vi "TryUpdateAnalogInputSample.vi"   [LabVIEW 2018]
uses:
  <vilib>/Platform/TimedLoop/XDataNode/timing_clust.ctl
  <vilib>/Platform/TimedLoop/XDataNode/nitl_modes.ctl
  <vilib>/Platform/TimedLoop/XDataNode/wakeup.ctl
  Telemetry/TelemetryDataTypes.ctl
  Telemetry/TelemetryUpdateModes.ctl
  Telemetry/TelemetryFields.ctl
  <vilib>/rvi/Emulation/niFpgaEmulationIsFPGAContextNoSignature.vi
  <vilib>/rvi/Emulation/niFpgaSctlEmulationGetInTimedLoop.vi
  <vilib>/rvi/errors/niFpgaSetErrorForExecOnDevCompSimple.vi
  <vilib>/rvi/eio/common/nirviEmuReportErrorAndStop.vi
  <vilib>/rvi/DataTransferAndStorage/Container/Common/niFpgaContainerGetUniqueNameForEmu.vi
  <vilib>/rvi/FIFO/Fifo_Resource/nirvififoEmulationSetSize.vi
  <vilib>/rvi/FIFO/Fifo_Resource/nirviFifoEmulationQueueMgr.vi
  <instcachedir>/0/nirviFifoEmulationQueueMgr_E5CAEC123FF24DC58D834DCA3CDAA9B5.lvgen/nirviFifoEmulationQueueMgr_E5CAEC123FF24DC58D834DCA3CDAA9B5_025.vi
  <vilib>/Utility/error.llb/Clear Errors.vi
  <vilib>/rvi/FIFO/Fifo_Resource/nirvififoEmulationCreateLock.vi
  <vilib>/rvi/Emulation/niFpgaProcessEmulError.vi
  <vilib>/rvi/FIFO/Fifo_Resource/nirvififoEmulationObtainLock.vi
  <vilib>/rvi/FIFO/Fifo_Resource/nirvififoEmulationReleaseLock.vi
  <vilib>/rvi/occurrence/nirviWaitOnOccurrenceBase.vi
  <vilib>/rvi/errors/nirviReportUnexpectedCaseInternalError.vi
  <vilib>/rvi/errors/nirviReportUnexpectedCaseInternalError (U32).vi
  <vilib>/rvi/Emulation/niFpgaEmulationReportErrorSimple.vi
  <vilib>/rvi/Emulation/niFpgaGetClockAttributes.vi
  <vilib>/rvi/Emulation/niFpgaCriticalErrorInLSC.vi
  <instcachedir>/0/nirviFifoEmulationQueueMgr_E5CAEC123FF24DC58D834DCA3CDAA9B5.lvgen/nirviFifoEmulationQueueMgr_E5CAEC123FF24DC58D834DCA3CDAA9B5_022.vi
  <vilib>/rvi/FIFO/Fifo_Resource/nirvififoEmulationDetermineInputValidOut.vi
  <instcachedir>/0/nirviFifoEmulationQueueMgr_E5CAEC123FF24DC58D834DCA3CDAA9B5.lvgen/nirviFifoEmulationQueueMgr_E5CAEC123FF24DC58D834DCA3CDAA9B5_023.vi
  <vilib>/rvi/Memory/Memory_Emulation/niFpgaMemoryEmulationCacheClearOnFirstRun.vi
  <vilib>/rvi/Memory/Memory_Emulation/nirvimemoryEmulationManagerCache_MakeExclusive.vi
  <vilib>/rvi/Memory/Memory_Emulation/niFpgaMemoryEmulationValidateCache.vi
  <vilib>/rvi/Memory/Memory_Emulation/nirvimemoryEmulationManagerCache_InsertValue.vi
  <vilib>/rvi/Memory/Memory_Emulation/nirvimemoryEmulationManagerCache_ReleaseExclusive.vi
  <vilib>/rvi/Memory/Memory_Emulation/nirvimemoryEmulationManagerCache_GetValue.vi
  <vilib>/rvi/Memory/Memory_Emulation/nirvimemoryEmulationManagerCache_SetValue.vi
  <instcachedir>/0/nirviFifoEmulationQueueMgr_E5CAEC123FF24DC58D834DCA3CDAA9B5.lvgen/nirviFifoEmulationQueueMgr_E5CAEC123FF24DC58D834DCA3CDAA9B5_002.vi
  <vilib>/rvi/DataTransferAndStorage/Container/XNode/niFpgaContainer.xnode
  <vilib>/rvi/FIFO/Fifo_Resource/nirvififoEmulationRead.vi
  <vilib>/Platform/TimedLoop/XDataNode/XDataNode.xnode
  <vilib>/rvi/FIFO/Fifo_Resource/nirvififoEmulationWrite.vi
  <vilib>/rvi/DataTransferAndStorage/Register/Emulation/niFpgaRegisterEmulation.vi
  <vilib>/Platform/TimedLoop/XDataNode/XDNodeRunTimeDep.lvlib
types:
  T1 = cluster{"Sample":u64, "Timestamp":u64, "Raw1":sgl, "Raw2":sgl, "Raw3":sgl, "Raw4":sgl, "Raw5":sgl, "Raw6":sgl, "Raw7":sgl, "Raw8":sgl, "Raw9":sgl, "Raw10":sgl, "Raw11":sgl, "Raw12":sgl, "Raw13":sgl, "Raw14":sgl, "Raw15":sgl, "Raw16":sgl}
  T2 = typedef "TelemetryFields.ctl" = enum16{"None", "AnalogInputSampleCount", "AnalogInputSampleTimestamp", "AnalogInputRaw1", "AnalogInputRaw2", "AnalogInputRaw3", "AnalogInputRaw4", "AnalogInputRaw5", "AnalogInputRaw6", "AnalogInputRaw7", "AnalogInputRaw8", "AnalogInputRaw9", "AnalogInputRaw10", "AnalogInputRaw11", "AnalogInputRaw12", "AnalogInputRaw13", "AnalogInputRaw14", "AnalogInputRaw15", "AnalogInputRaw16", "DigitalInputSampleCount", "DigitalInputSampleTimestamp", "DigitalInputStates", "ThermocoupleSampleCount", "ThermocoupleSampleTimestamp", "ThermocoupleRaw1", "ThermocoupleRaw2", "ThermocoupleRaw3", "ThermocoupleRaw4", "ThermocoupleRaw5", "ThermocoupleRaw6", "ThermocoupleRaw7", "ThermocoupleRaw8", "ThermocoupleRaw9", "ThermocoupleRaw10", "ThermocoupleRaw11", "ThermocoupleRaw12", "ThermocoupleRaw13", "ThermocoupleRaw14", "ThermocoupleRaw15", "ThermocoupleRaw16", "WindSensorTxBytes", "WindSensorTxFrames", "WindSensorRxBytes", "WindSensorRxFrames", "WindSensorErrorTimestamp", "WindSensorErrorCode", "WindSensorSampleTimestamp", "WindSensorXRaw", "WindSensorYRaw", "WindSensorZRaw", "WindSensorSonicTempRaw", "WindSensorDiagWord", "WindSensorRecordCount", "FlowSensorTxBytes", "FlowSensorTxFrames", "FlowSensorRxBytes", "FlowSensorRxFrames", "FlowSensorErrorTimestamp", "FlowSensorErrorCode", "FlowSensorSampleTimestamp", "FlowSensorSignalStrength", "FlowSensorFlowRate", "FlowSensorNetTotalizer", "FlowSensorPositiveTotalizer", "FlowSensorNegativeTotalizer", "FlowSensorTemperature1", "FlowSensorTemperature2", "VFDTxBytes", "VFDTxFrames", "VFDRxBytes", "VFDRxFrames", "VFDErrorTimestamp", "VFDErrorCode", "VFDSampleTimestamp", "VFDVelocityBits", "VFDDiagnosticCode", "VFDFrequencyCommand", "VFDOutputFrequency", "VFDOutputCurrent", "VFDDCBusVoltage", "VFDOutputVoltage"}
  T3 = typedef "TelemetryUpdateModes.ctl" = enum8{"=", "+", "-", "|"}
  T4 = typedef "TelemetryDataTypes.ctl" = enum8{"U8", "U16", "U32", "U64", "I8", "I16", "I32", "I64", "SGL"}
  T5 = typedef "XDNodeRunTimeDep.lvlib/timing_clust.ctl" = cluster{"Expected End [f-1]":u64, "Actual End [f-1]":u64, "Finished Late? [f-1]":bool, "Expected End [i-1]":u64, "Actual End [i-1]":u64, "Finished Late? [i-1]":bool, "Expected Start [i]":u64, "Actual Start [i]":u64, "Expected Start [f]":u64, "Actual Start [f]":u64, "Source Name":string, "Structure Name":string, "Period":i64, "Deadline":i64, "Offset":i64, "Start":i64, "Priority":i32, "Timeout":i32, "Mode":T6, "Wakeup Reason":T7, "Error":errorcluster, "Source Type":string, "Secondary Source Type":string, "Global End Time":u64, "Global Start Time":u64, "Frame Duration":u64, "Iteration Duration":u64, "Assigned CPU":i32, "I/O Scan Engine Mode":u32}
  T6 = typedef "XDNodeRunTimeDep.lvlib/nitl_modes.ctl" = enum32{"No Change", "Process missed periods, maintain original phase", "Discard missed periods, maintain original phase", "Process missed periods, ignore original phase", "Discard missed periods, ignore original phase"}
  T7 = typedef "XDNodeRunTimeDep.lvlib/wakeup.ctl" = enum32{"Normal", "Aborted", "Asynchronous wakeup", "Timing source error", "Timed loop error", "Timeout"}
  T8 = typedef "TelemetryUpdateData.ctl" = cluster{"DataType":T4, "Mode":T3, "Field":T2, "Data":u64}
  T9 = typedef "TelemetryUpdateDataSGL.ctl" = cluster{"Mode":T3, "Field":T2, "Data":sgl}
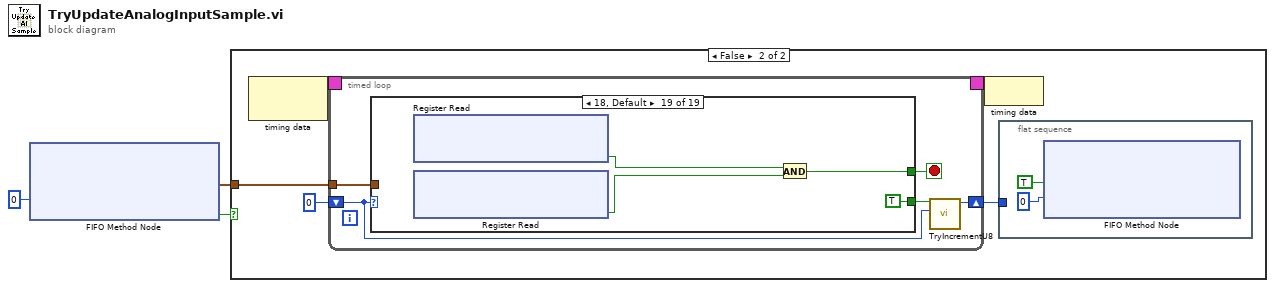
[diagram p0: block diagram]
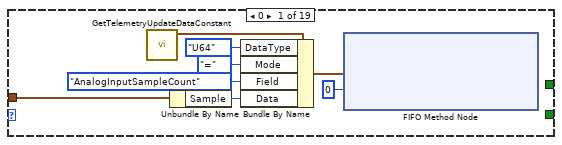
[diagram p3: hidden frame]
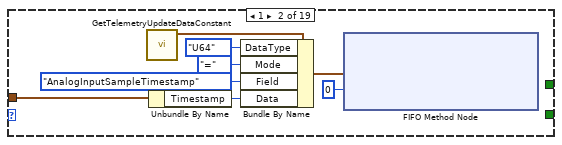
[diagram p4: hidden frame]
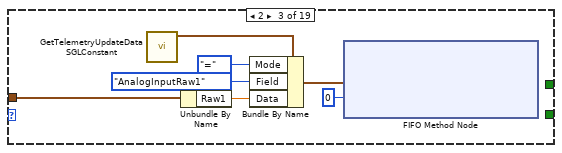
[diagram p5: hidden frame]
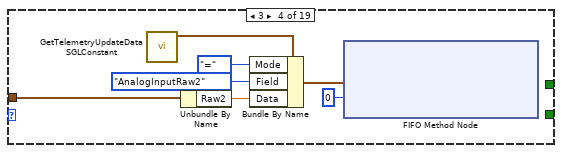
[diagram p6: hidden frame]
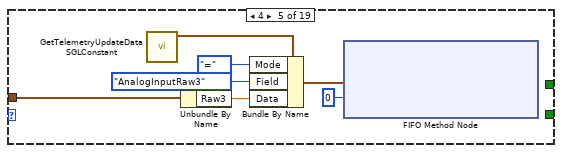
[diagram p7: hidden frame]
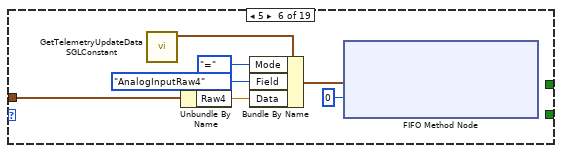
[diagram p8: hidden frame]
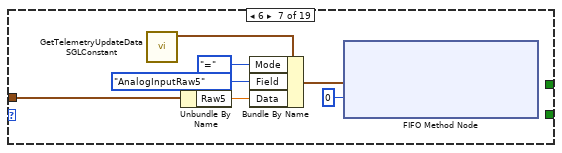
[diagram p9: hidden frame]
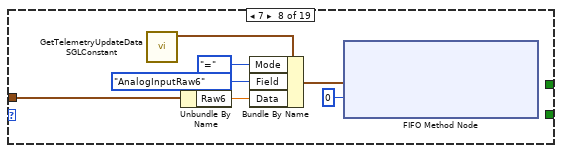
[diagram p10: hidden frame]
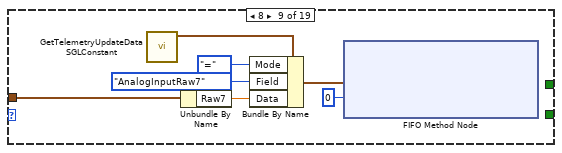
[diagram p11: hidden frame]
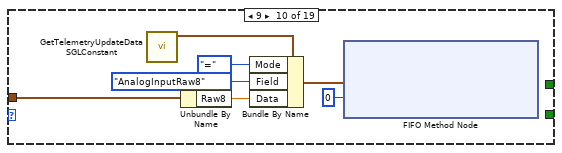
[diagram p12: hidden frame]
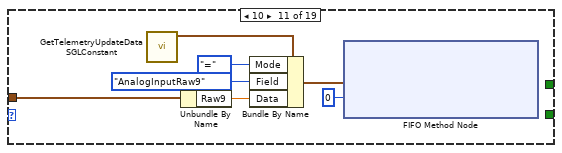
[diagram p13: hidden frame]
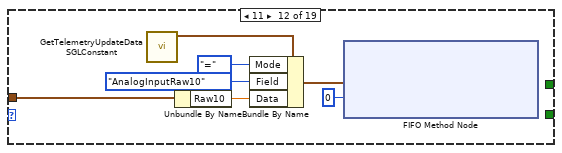
[diagram p14: hidden frame]
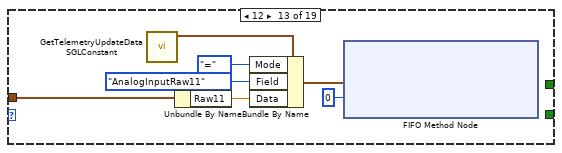
[diagram p15: hidden frame]
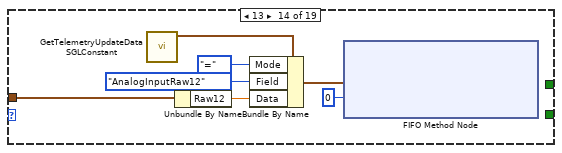
[diagram p16: hidden frame]
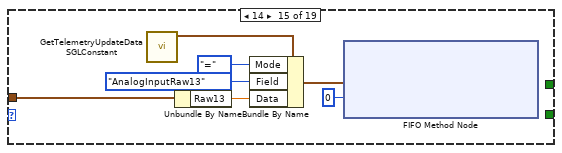
[diagram p17: hidden frame]
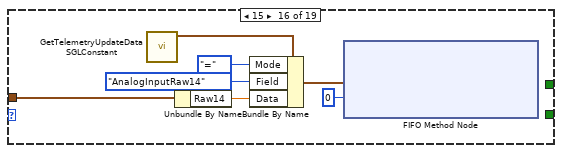
[diagram p18: hidden frame]
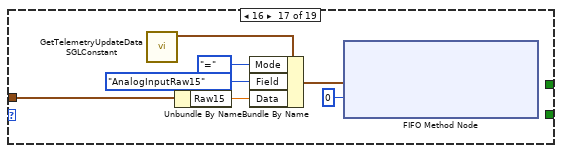
[diagram p19: hidden frame]
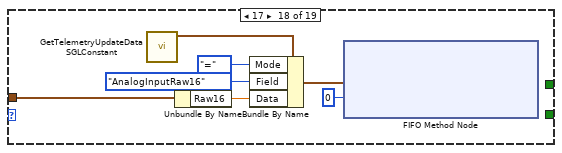
[diagram p20: hidden frame]
diagram:
  n1 = xnode ("FIFO Method Node")("Timeout"=0) -> ("Element"=w2:T1, "Timed Out?"=w3:bool)  [unwired: 1 in, 1 out]
  n2 = case shown="False" w3 {
    tunnel: w2 -> [_ w8]
    frame True {
    }
    frame False {
      n3 = node-c288() -> (w7:T5)  [unwired: 1 in]
      n4 = timed-loop {
        tunnel: w8 -> [w13]
        timing: w7 -> [_]
        timing-out: [_] -> w6
        shift-right: [w11] -> w4
        shift-left: u8 0 -> [w10]
        stop <- w12 stop-if-true
        # "Move Data to Memory"
        n5 = case shown="18, Default" w10 {
          tunnel: w13 -> [w15 w23 w31 w38 w45 w52 w59 w66 w73 w80 w87 w94 w101 w108 w115 w122 w129 w136 _]
          tunnel: [_ _ _ _ _ _ _ _ _ _ _ _ _ _ _ _ _ _ w145] -> w12
          tunnel: [_ _ _ _ _ _ _ _ _ _ _ _ _ _ _ _ _ _ TRUE] -> w9
          frame 0 {
            n6 = call "GetTelemetryUpdateDataConstant.vi"() -> ("TelemetryUpdateData"=w21:T8)  [unwired: 11 in]
            n7 = Unbundle By Name(w15) -> ("Sample"=w14:u64)
            n8 = Bundle By Name(cluster=w21, "DataType"=TelemetryDataTypes."U64" ("TelemetryDataTypes"), "Mode"=TelemetryUpdateModes."=" ("TelemetryUpdateModes"), "Field"=TelemetryFields."AnalogInputSampleCount" ("TelemetryFields"), "Data"=w14) -> (w19:T8)
            n9 = xnode ("FIFO Method Node")("Element"=w19, "Timeout"=0) -> ()  [unwired: 1 in, 2 out]
          }
          frame 1 {
            n10 = call "GetTelemetryUpdateDataConstant.vi"() -> ("TelemetryUpdateData"=w29:T8)  [unwired: 11 in]
            n11 = Unbundle By Name(w23) -> ("Timestamp"=w22:u64)
            n12 = Bundle By Name(cluster=w29, "DataType"=TelemetryDataTypes."U64" ("TelemetryDataTypes"), "Mode"=TelemetryUpdateModes."=" ("TelemetryUpdateModes"), "Field"=TelemetryFields."AnalogInputSampleTimestamp" ("TelemetryFields"), "Data"=w22) -> (w27:T8)
            n13 = xnode ("FIFO Method Node")("Element"=w27, "Timeout"=0) -> ()  [unwired: 1 in, 2 out]
          }
          frame 2 {
            n14 = call "GetTelemetryUpdateDataSGLConstant.vi"() -> ("TelemetryUpdateDataSGL"=w36:T9)  [unwired: 11 in]
            n15 = Unbundle By Name(w31) -> ("Raw1"=w30:sgl)
            n16 = Bundle By Name(cluster=w36, "Mode"=TelemetryUpdateModes."=" ("TelemetryUpdateModes"), "Field"=TelemetryFields."AnalogInputRaw1" ("TelemetryFields"), "Data"=w30) -> (w34:T9)
            n17 = xnode ("FIFO Method Node")("Element"=w34, "Timeout"=0) -> ()  [unwired: 1 in, 2 out]
          }
          frame 3 {
            n18 = call "GetTelemetryUpdateDataSGLConstant.vi"() -> ("TelemetryUpdateDataSGL"=w43:T9)  [unwired: 11 in]
            n19 = Unbundle By Name(w38) -> ("Raw2"=w37:sgl)
            n20 = Bundle By Name(cluster=w43, "Mode"=TelemetryUpdateModes."=" ("TelemetryUpdateModes"), "Field"=TelemetryFields."AnalogInputRaw2" ("TelemetryFields"), "Data"=w37) -> (w41:T9)
            n21 = xnode ("FIFO Method Node")("Element"=w41, "Timeout"=0) -> ()  [unwired: 1 in, 2 out]
          }
          frame 4 {
            n22 = call "GetTelemetryUpdateDataSGLConstant.vi"() -> ("TelemetryUpdateDataSGL"=w50:T9)  [unwired: 11 in]
            n23 = Unbundle By Name(w45) -> ("Raw3"=w44:sgl)
            n24 = Bundle By Name(cluster=w50, "Mode"=TelemetryUpdateModes."=" ("TelemetryUpdateModes"), "Field"=TelemetryFields."AnalogInputRaw3" ("TelemetryFields"), "Data"=w44) -> (w48:T9)
            n25 = xnode ("FIFO Method Node")("Element"=w48, "Timeout"=0) -> ()  [unwired: 1 in, 2 out]
          }
          frame 5 {
            n26 = call "GetTelemetryUpdateDataSGLConstant.vi"() -> ("TelemetryUpdateDataSGL"=w57:T9)  [unwired: 11 in]
            n27 = Unbundle By Name(w52) -> ("Raw4"=w51:sgl)
            n28 = Bundle By Name(cluster=w57, "Mode"=TelemetryUpdateModes."=" ("TelemetryUpdateModes"), "Field"=TelemetryFields."AnalogInputRaw4" ("TelemetryFields"), "Data"=w51) -> (w55:T9)
            n29 = xnode ("FIFO Method Node")("Element"=w55, "Timeout"=0) -> ()  [unwired: 1 in, 2 out]
          }
          frame 6 {
            n30 = call "GetTelemetryUpdateDataSGLConstant.vi"() -> ("TelemetryUpdateDataSGL"=w64:T9)  [unwired: 11 in]
            n31 = Unbundle By Name(w59) -> ("Raw5"=w58:sgl)
            n32 = Bundle By Name(cluster=w64, "Mode"=TelemetryUpdateModes."=" ("TelemetryUpdateModes"), "Field"=TelemetryFields."AnalogInputRaw5" ("TelemetryFields"), "Data"=w58) -> (w62:T9)
            n33 = xnode ("FIFO Method Node")("Element"=w62, "Timeout"=0) -> ()  [unwired: 1 in, 2 out]
          }
          frame 7 {
            n34 = call "GetTelemetryUpdateDataSGLConstant.vi"() -> ("TelemetryUpdateDataSGL"=w71:T9)  [unwired: 11 in]
            n35 = Unbundle By Name(w66) -> ("Raw6"=w65:sgl)
            n36 = Bundle By Name(cluster=w71, "Mode"=TelemetryUpdateModes."=" ("TelemetryUpdateModes"), "Field"=TelemetryFields."AnalogInputRaw6" ("TelemetryFields"), "Data"=w65) -> (w69:T9)
            n37 = xnode ("FIFO Method Node")("Element"=w69, "Timeout"=0) -> ()  [unwired: 1 in, 2 out]
          }
          frame 8 {
            n38 = call "GetTelemetryUpdateDataSGLConstant.vi"() -> ("TelemetryUpdateDataSGL"=w78:T9)  [unwired: 11 in]
            n39 = Unbundle By Name(w73) -> ("Raw7"=w72:sgl)
            n40 = Bundle By Name(cluster=w78, "Mode"=TelemetryUpdateModes."=" ("TelemetryUpdateModes"), "Field"=TelemetryFields."AnalogInputRaw7" ("TelemetryFields"), "Data"=w72) -> (w76:T9)
            n41 = xnode ("FIFO Method Node")("Element"=w76, "Timeout"=0) -> ()  [unwired: 1 in, 2 out]
          }
          frame 9 {
            n42 = call "GetTelemetryUpdateDataSGLConstant.vi"() -> ("TelemetryUpdateDataSGL"=w85:T9)  [unwired: 11 in]
            n43 = Unbundle By Name(w80) -> ("Raw8"=w79:sgl)
            n44 = Bundle By Name(cluster=w85, "Mode"=TelemetryUpdateModes."=" ("TelemetryUpdateModes"), "Field"=TelemetryFields."AnalogInputRaw8" ("TelemetryFields"), "Data"=w79) -> (w83:T9)
            n45 = xnode ("FIFO Method Node")("Element"=w83, "Timeout"=0) -> ()  [unwired: 1 in, 2 out]
          }
          frame 10 {
            n46 = call "GetTelemetryUpdateDataSGLConstant.vi"() -> ("TelemetryUpdateDataSGL"=w92:T9)  [unwired: 11 in]
            n47 = Unbundle By Name(w87) -> ("Raw9"=w86:sgl)
            n48 = Bundle By Name(cluster=w92, "Mode"=TelemetryUpdateModes."=" ("TelemetryUpdateModes"), "Field"=TelemetryFields."AnalogInputRaw9" ("TelemetryFields"), "Data"=w86) -> (w90:T9)
            n49 = xnode ("FIFO Method Node")("Element"=w90, "Timeout"=0) -> ()  [unwired: 1 in, 2 out]
          }
          frame 11 {
            n50 = call "GetTelemetryUpdateDataSGLConstant.vi"() -> ("TelemetryUpdateDataSGL"=w99:T9)  [unwired: 11 in]
            n51 = Unbundle By Name(w94) -> ("Raw10"=w93:sgl)
            n52 = Bundle By Name(cluster=w99, "Mode"=TelemetryUpdateModes."=" ("TelemetryUpdateModes"), "Field"=TelemetryFields."AnalogInputRaw10" ("TelemetryFields"), "Data"=w93) -> (w97:T9)
            n53 = xnode ("FIFO Method Node")("Element"=w97, "Timeout"=0) -> ()  [unwired: 1 in, 2 out]
          }
          frame 12 {
            n54 = call "GetTelemetryUpdateDataSGLConstant.vi"() -> ("TelemetryUpdateDataSGL"=w106:T9)  [unwired: 11 in]
            n55 = Unbundle By Name(w101) -> ("Raw11"=w100:sgl)
            n56 = Bundle By Name(cluster=w106, "Mode"=TelemetryUpdateModes."=" ("TelemetryUpdateModes"), "Field"=TelemetryFields."AnalogInputRaw11" ("TelemetryFields"), "Data"=w100) -> (w104:T9)
            n57 = xnode ("FIFO Method Node")("Element"=w104, "Timeout"=0) -> ()  [unwired: 1 in, 2 out]
          }
          frame 13 {
            n58 = call "GetTelemetryUpdateDataSGLConstant.vi"() -> ("TelemetryUpdateDataSGL"=w113:T9)  [unwired: 11 in]
            n59 = Unbundle By Name(w108) -> ("Raw12"=w107:sgl)
            n60 = Bundle By Name(cluster=w113, "Mode"=TelemetryUpdateModes."=" ("TelemetryUpdateModes"), "Field"=TelemetryFields."AnalogInputRaw12" ("TelemetryFields"), "Data"=w107) -> (w111:T9)
            n61 = xnode ("FIFO Method Node")("Element"=w111, "Timeout"=0) -> ()  [unwired: 1 in, 2 out]
          }
          frame 14 {
            n62 = call "GetTelemetryUpdateDataSGLConstant.vi"() -> ("TelemetryUpdateDataSGL"=w120:T9)  [unwired: 11 in]
            n63 = Unbundle By Name(w115) -> ("Raw13"=w114:sgl)
            n64 = Bundle By Name(cluster=w120, "Mode"=TelemetryUpdateModes."=" ("TelemetryUpdateModes"), "Field"=TelemetryFields."AnalogInputRaw13" ("TelemetryFields"), "Data"=w114) -> (w118:T9)
            n65 = xnode ("FIFO Method Node")("Element"=w118, "Timeout"=0) -> ()  [unwired: 1 in, 2 out]
          }
          frame 15 {
            n66 = call "GetTelemetryUpdateDataSGLConstant.vi"() -> ("TelemetryUpdateDataSGL"=w127:T9)  [unwired: 11 in]
            n67 = Unbundle By Name(w122) -> ("Raw14"=w121:sgl)
            n68 = Bundle By Name(cluster=w127, "Mode"=TelemetryUpdateModes."=" ("TelemetryUpdateModes"), "Field"=TelemetryFields."AnalogInputRaw14" ("TelemetryFields"), "Data"=w121) -> (w125:T9)
            n69 = xnode ("FIFO Method Node")("Element"=w125, "Timeout"=0) -> ()  [unwired: 1 in, 2 out]
          }
          frame 16 {
            n70 = call "GetTelemetryUpdateDataSGLConstant.vi"() -> ("TelemetryUpdateDataSGL"=w134:T9)  [unwired: 11 in]
            n71 = Unbundle By Name(w129) -> ("Raw15"=w128:sgl)
            n72 = Bundle By Name(cluster=w134, "Mode"=TelemetryUpdateModes."=" ("TelemetryUpdateModes"), "Field"=TelemetryFields."AnalogInputRaw15" ("TelemetryFields"), "Data"=w128) -> (w132:T9)
            n73 = xnode ("FIFO Method Node")("Element"=w132, "Timeout"=0) -> ()  [unwired: 1 in, 2 out]
          }
          frame 17 {
            n74 = call "GetTelemetryUpdateDataSGLConstant.vi"() -> ("TelemetryUpdateDataSGL"=w141:T9)  [unwired: 11 in]
            n75 = Unbundle By Name(w136) -> ("Raw16"=w135:sgl)
            n76 = Bundle By Name(cluster=w141, "Mode"=TelemetryUpdateModes."=" ("TelemetryUpdateModes"), "Field"=TelemetryFields."AnalogInputRaw16" ("TelemetryFields"), "Data"=w135) -> (w139:T9)
            n77 = xnode ("FIFO Method Node")("Element"=w139, "Timeout"=0) -> ()  [unwired: 1 in, 2 out]
          }
          frame 18, Default {
            n78 = xnode ("Register Read")() -> ("Data"=w143:bool)  [unwired: 1 in, 1 out]
            n79 = xnode "Register Read"() -> ("Data"=w144:bool)  [unwired: 1 in, 1 out]
            n80 = And(x=w143, y=w144) -> (x .and. y?=w145:bool)
          }
        }
        n81 = call "TryIncrementU8.vi"("In"=w10, "DontInc"=w9) -> ("Out"=w11:u8)  [unwired: 9 in]
      }
      n82 = node-c288(w6) -> ()
      n83 = flat-sequence {
        tunnel: w4 -> [_]
        frame #0 {
          n84 = xnode ("FIFO Method Node")("Element"=TRUE, "Timeout"=0) -> ()  [unwired: 1 in, 2 out]
        }
      }
    }
  }
